vi "CallSystemForms.vi"(8 "error in (no error)":errorcluster, 11 "Path In":path) -> (0 "error out":errorcluster, 2 "ButtonPressed":i32(ring) items=["None", "OK", "Cancel", "Abort", "Retry", "Ignore", "Yes", "No"], 3 "Path Out":path)   [LabVIEW 2022 SP3]
uses:
  System.Windows.Forms
panel:
  # "NOTE:"
  # "File » VI Properties,,, » Execution » Preferred Execution System: user interface"
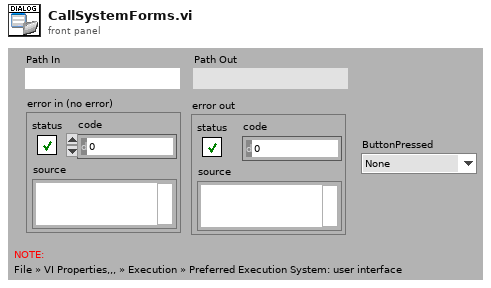
[diagram p1: front panel]
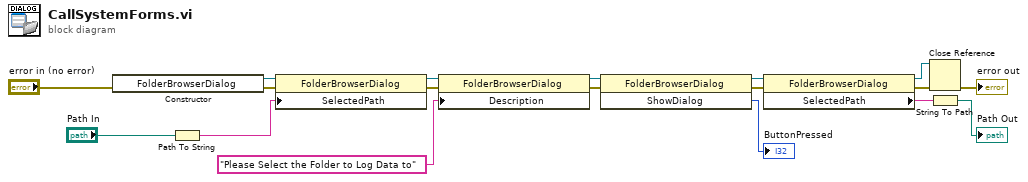
[diagram p0: block diagram]
diagram:
  n1 = constructor class="FolderBrowserDialog"(error in="error in (no error)") -> (reference out=w4:refnum<k24>, error out=w2:errorcluster)  [unwired: 2 in, 1 out]
  n2 = Path To String(path="Path In") -> (string=w5:string)
  n3 = property class="FolderBrowserDialog"(reference=w4, error in=w2, "SelectedPath"=w5) -> (reference out=w3:refnum<k24>, error out=w1:errorcluster)
  n4 = property class="FolderBrowserDialog"(reference=w3, error in=w1, "Description"="Please Select the Folder to Log Data to") -> (reference out=w17:refnum<k24>, error out=w16:errorcluster)
  n5 = invoke class="FolderBrowserDialog" method="ShowDialog"(reference=w17, error in=w16) -> (reference out=w15:refnum<k24>, error out=w14:errorcluster, "ShowDialog"=→"ButtonPressed":i32)  [unwired: 1 in]
  n6 = property class="FolderBrowserDialog"(reference=w15, error in=w14) -> (reference out=w11:refnum<k24>, error out=w12:errorcluster, "SelectedPath"=w13:string)
  n7 = Close Reference(reference=w11, error in (no error)=w12) -> (error out=→"error out":errorcluster)
  n8 = String To Path(string=w13) -> (path=→"Path Out":path)
